vi "LINC Parse Handshake.vi"(10 "GUID bitoffset":i32, 11 "command packet":string) -> (1 "error source":string, 2 "GUID":string, 3 "command data":string)   [LabVIEW 2018, in "STEPkgDriver_LINC.lvlib"]
uses:
  STEPkgDriver_LINC.lvlib
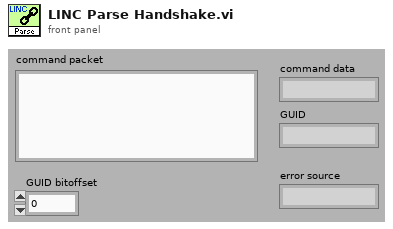
[diagram p1: front panel]
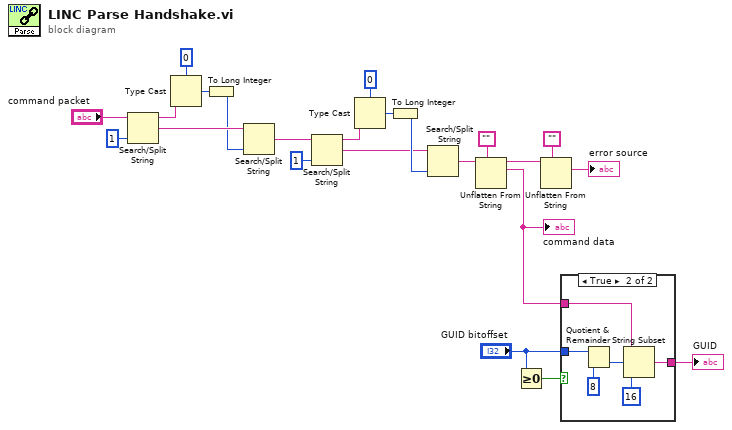
[diagram p0: block diagram]
diagram:
  n1 = Search/Split String(string="command packet", offset (0)=1) -> (substring before match=w21:string, match + rest of string=w18:string)  [unwired: 1 in, 1 out]
  n2 = Type Cast(type=u8 0, x=w21) -> (*(type *) &x=w19:u8)
  n3 = To Long Integer(number=w19) -> (32bit integer=w17:i32)
  n4 = Search/Split String(string=w18, offset (0)=w17) -> (match + rest of string=w10:string)  [unwired: 1 in, 2 out]
  n5 = Search/Split String(string=w10, offset (0)=1) -> (substring before match=w12:string, match + rest of string=w15:string)  [unwired: 1 in, 1 out]
  n6 = Type Cast(type=u8 0, x=w12) -> (*(type *) &x=w14:u8)
  n7 = To Long Integer(number=w14) -> (32bit integer=w16:i32)
  n8 = Search/Split String(string=w15, offset (0)=w16) -> (match + rest of string=w9:string)  [unwired: 1 in, 2 out]
  n9 = Unflatten From String(type="", binary string=w9) -> (rest of the binary string=w2:string, value=w6:string)  [unwired: 3 in, 1 out]
  "command data" <- w6
  n10 = Greater Or Equal To 0?(x="GUID bitoffset") -> (x >= 0?=w7:bool)
  n11 = Unflatten From String(type="", binary string=w2) -> (value=→"error source":string)  [unwired: 3 in, 2 out]
  n12 = case shown="True" w7 {
    tunnel: w6 -> [_ w29]
    tunnel: "GUID bitoffset" -> [_ w28]
    tunnel: [_ w24] -> w5
    frame False {
    }
    frame True {
      n13 = Quotient & Remainder(x=w28, y=8) -> (floor(x/y)=w26:i32)  [unwired: 1 out]
      n14 = String Subset(string=w29, offset (0)=w26, length (rest)=16 ("length (rest)")) -> (substring=w24:string)
    }
  }
  "GUID" <- w5
